vi "Memory.Pointer.Numeric.New.vi"(8 "error in (no error)":errorcluster, 11 "power of 2":i16) -> (0 "error out":errorcluster, 3 "Numeric Pointer out":refnum<class "Memory.Pointer.Numeric.lvclass">)   [LabVIEW 2016, in "Memory.Pointer.Numeric.lvclass"]
uses:
  Memory.Pointer.Numeric.lvclass
  C:/Users/Ryan/Documents/Git/Sourcetree/LabVIEW-Memory-Manager/Source/Library/Classes/Pointer/Pointer.Void/Memory.Pointer.Void.lvclass
  Memory.Pointer.Numeric.lvclass/Memory.Pointer.Numeric.ctl
  Pointer.Void/Memory.Pointer.Void.lvclass/Memory.Pointer.Void.ctl
  Pointer.Void/Methods/Memory.Pointer.Set Size.vi
  Pointer.Void/Methods/Memory.Pointer.Set Address.vi
  Pointer.Void/Methods/Memory.Pointer.Get Size.vi
  Pointer.Void/Memory.Pointer.Void.lvclass
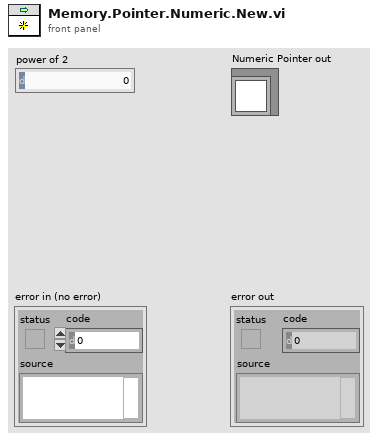
[diagram p1: front panel]
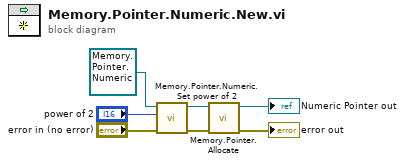
[diagram p0: block diagram]
diagram:
  n1 = call "Memory.Pointer.Numeric.Set power of 2.vi"("error in (no error)"="error in (no error)", "power of 2"="power of 2", "Numeric Pointer in"=refnum<class "Memory.Pointer.Numeric.lvclass"> refnum) -> ("error out"=w4:errorcluster, "Numeric Pointer out"=w5:refnum<class "Memory.Pointer.Numeric.lvclass">)  [unwired: 7 in]
  n2 = call "Memory.Pointer.Allocate.vi"("error in (no error)"=w4, "Pointer in"=w5) -> ("error out"=→"error out":errorcluster, "Pointer out"=→"Numeric Pointer out":refnum<class "Memory.Pointer.Numeric.lvclass">)  [unwired: 7 in, 1 out]
